vi "prepare v2.vi"(8 "error in (no error)":errorcluster, 10 "zSql":string, 11 "db":u64) -> (0 "error out":errorcluster, 1 "pzTail":string, 2 "ppStmt out":u64)   [LabVIEW 2020, in "sqlite3.lvlib"]
uses:
  sqlite3.lvlib
  errstr.vi
  bin/sqlite3_64.dll
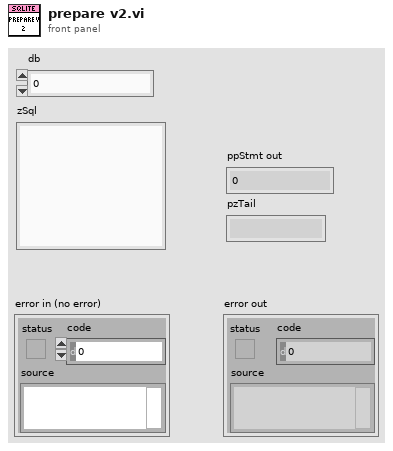
[diagram p1: front panel]
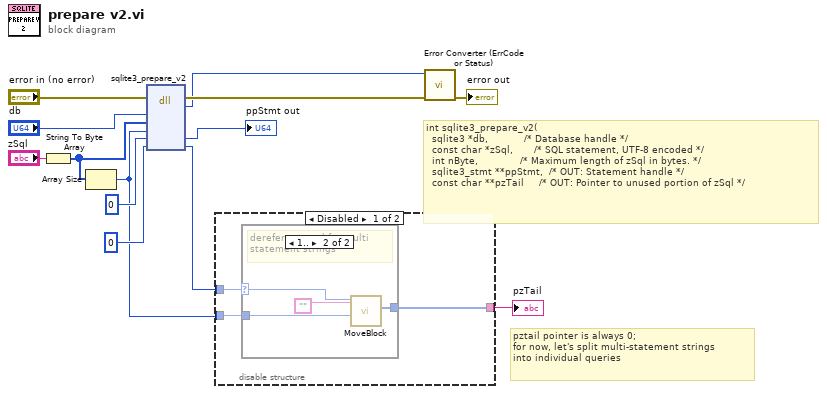
[diagram p0: block diagram]
diagram:
  # "pztail pointer is always 0;\nfor now, let's split multi-statement strings\ninto individual queries"
  # "int sqlite3_prepare_v2(\n  sqlite3 *db,            /* Database handle */\n  const char *zSql,       /* SQL statement, UTF-8 encoded */\n  int nByte,              /* Maximum length of zSql in bytes. */\n  sqlite3_stmt **ppStmt,  /* OUT: Statement handle */\n  const char **pzTail     /* OUT: Pointer to unused portion of zSql */"
  n1 = String To Byte Array(string="zSql") -> (unsigned byte array=w8:u8[])
  n2 = Array Size(array=w8) -> (size(s)=w3:i32)
  n3 = dll-call lib="D:/Project/Labview-Projects/database-configuration/externals/sqlite3/Source/bin/sqlite3_*.dll" fn="sqlite3_prepare_v2"(error in="error in (no error)", "db"="db", "zSql"=w8, "nByte"=w3, "ppStmt"=u64 0, "pzTail"=u64 0) -> (error out=w11:errorcluster, "return type"=w7:i32, "ppStmt"=→"ppStmt out":u64, "pzTail"=w4:u64)  [unwired: 5 in, 1 out]
  n4 = disable-structure shown="Disabled" {
    disable-tunnel: w4 -> [w16 _]
    disable-tunnel: w3 -> [w15 _]
    disable-tunnel: [w14 _] -> w2
    frame Disabled {
      n5 = case shown="1.." w16 {
        selector: w16 -> [_ w20]
        tunnel: w15 -> [_ w18]
        tunnel: [_ w17] -> w14
        frame 0, Default {
          # "null pointer\nfor single statements"
        }
        frame 1.. {
          # "dereference sql for multi\nstatement strings"
          n6 = call "MoveBlock.vi"("size"=w18, "destination (type)"="", "Address (pointer)"=w20) -> ("Value"=w17:u8[])  [unwired: 7 in, 1 out]
        }
      }
    }
    frame Enabled {
    }
  }
  "pzTail" <- w2
  n7 = call "Error Converter (ErrCode or Status).vi"("error in (no error)"=w11, "error code"=w7) -> ("error out"=→"error out":errorcluster)  [unwired: 9 in]
